vi "DAQ Rack AI Read (Dunk Tank).vi"(10 "Channel to Cal":u16(ring)=16 items=["AI-00", "AI-01", "AI-02", "AI-03", "AI-04", "AI-05", "AI-06", "AI-07", "AI-08", "AI-09", "AI-10", "AI-11", "AI-12", "AI-13", "AI-14", "AI-15", "AI-16", "AI-17", "AI-18", "AI-19", "AI-20", "AI-21", "AI-22", "AI-23", "AI-24", "AI-25", "AI-26", "AI-27", "AI-28", "AI-29", "AI-30", "AI-31", "TC-00", "TC-01", "TC-02", "TC-03", "TC-04", "TC-05", "TC-06", "TC-07", "TC-08", "TC-09", "TC-10", "TC-11", "TC-12", "TC-13", "TC-14", "TC-15"], 11 "Device":tag) -> (3 "Data":dbl format="%0.2f")   [LabVIEW 2013]
uses:
  <vilib>/DAQmx/read.llb/DAQmx Read (Analog DBL 1Chan 1Samp).vi
  <vilib>/DAQmx/create/channels.llb/DAQmx Create Channel (AI-Voltage-Basic).vi
  <vilib>/DAQmx/miscellaneous.llb/DAQmx Fill In Error Info.vi
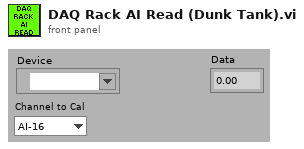
[diagram p1: front panel]
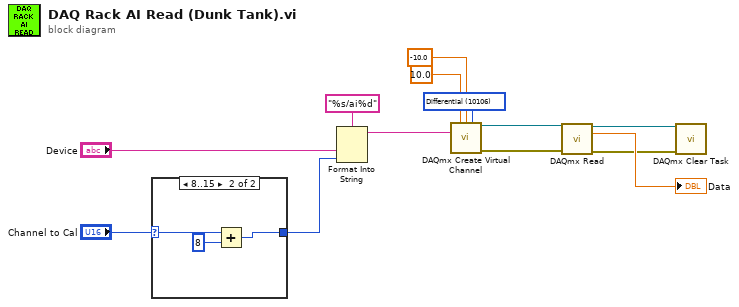
[diagram p0: block diagram]
diagram:
  w8 = 10106 items=["default"=-1, "RSE"=10083, "NRSE"=10078, "Differential"=10106, "Pseudodifferential"=12529] ("input terminal configuration")
  n1 = case shown="8..15" "Channel to Cal" {
    selector: "Channel to Cal" -> [w14 w17]
    tunnel: [w14 w15] -> w1
    frame 0..7, Default {
    }
    frame 8..15 {
      n2 = Add(x=w17, y=u16 8) -> (x+y=w15:u16)
    }
  }
  n3 = Format Into String(format string="%s/ai%d", "Device", w1) -> (resulting string=w10:string)  [unwired: 2 in, 1 out]
  n4 = call-poly <vilib>:"DAQmx Create Virtual Channel.vi"("maximum value"=10.0, "minimum value"=-10.0, "input terminal configuration"=w8, "physical channels"=w10) -> ("task out"=w7:refnum<k21>, "error out"=w6:errorcluster)  [unwired: 10 in]
  n5 = call-poly <vilib>:"DAQmx Read.vi"("task/channels in"=w7, "error in"=w6) -> ("task out"=w12:refnum<k21>, "data"=→"Data":dbl, "error out"=w11:errorcluster)  [unwired: 11 in]
  n6 = call <vilib>:"DAQmx Clear Task.vi"("task in"=w12, "error in"=w11) -> ()  [unwired: 13 in, 1 out]
